vi "Tag Source.vi"(8 "Error In":errorcluster) -> (0 "Error Out":errorcluster)   [LabVIEW 2018, in "Tests.lvlib" / "Nodes.lvlib"]
uses:
  Nodes.lvlib
  src/Toolkit/Low-Level/Nodes/Tag/Tag.lvclass
  <vilib>/addons/_JKI Toolkits/Caraya/classes/Test/Test.lvclass
  <vilib>/addons/_JKI Toolkits/Caraya/classes/Assert/Assert.lvclass
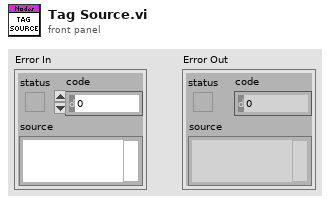
[diagram p1: front panel]
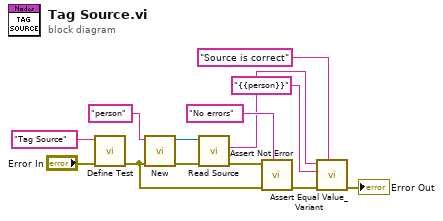
[diagram p0: block diagram]
diagram:
  n1 = call <vilib>:"Define Test.vi"("error in (no error)"="Error In", "Label (VI Title)"="Tag Source") -> ("error out"=w5:errorcluster)  [unwired: 9 in]
  n2 = call "New.vi"("Error In"=w5, "Key"="person") -> ("Error Out"=w2:errorcluster, "Tag"=w1:refnum<class "Tag.lvclass">)  [unwired: 8 in]
  n3 = call-dynamic "Read Source.vi"("Error In"=w2, "Node In"=w1) -> ("Error Out"=w9:errorcluster, "Source"=w8:string)  [unwired: 7 in, 1 out]
  n4 = call <vilib>:"Assert Not Error.vi"("Label"="No errors", "error in (no error)"=w5, "Not Error?"=w9) -> ("error out"=w11:errorcluster)  [unwired: 8 in]
  n5 = call <vilib>:"Assert Equal Value_Variant.vi"("Label"="Source is correct", "error in (no error)"=w11, "Y"="{{person}}" ("format string"), "X"=w8) -> ("error out"=→"Error Out":errorcluster)  [unwired: 7 in]
